vi "Downsample image.vi"(8 "error in (no error)":errorcluster, 10 "Original image":u16[][](array[numeric]), 11 "TomoConversion in":refnum<class "TomoConversion.lvclass">) -> (0 "error out":errorcluster, 2 "Downsampled image":u16[][](array[numeric]), 3 "TomoConversion out":refnum<class "TomoConversion.lvclass">)   [LabVIEW 2012, in "TomoConversion.lvclass"]
uses:
  TomoConversion.lvclass
  TomoConversion.lvclass/TomoConversion.ctl
  <vilib>/Analysis/baseanly.llb/Mean (DBL).vi
  <vilib>/Analysis/NI_AALBase.lvlib
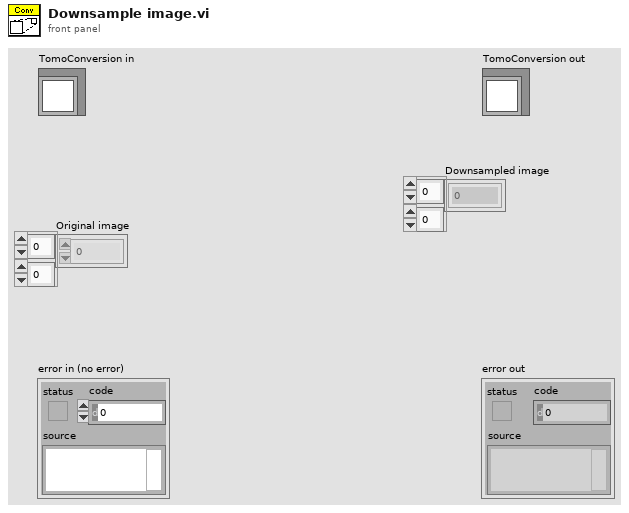
[diagram p1: front panel]
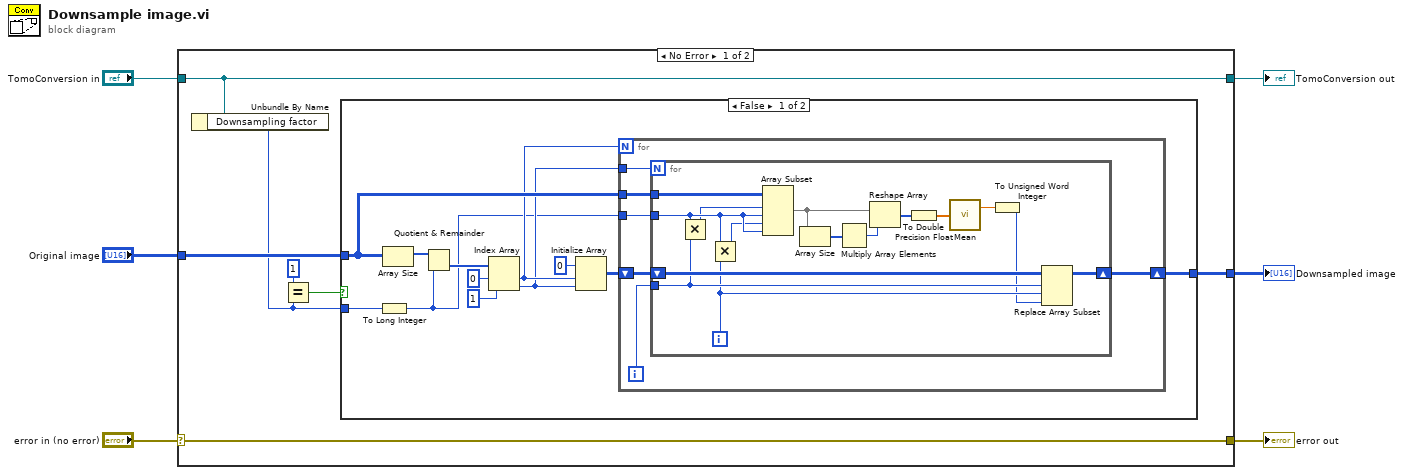
[diagram p0: block diagram]
diagram:
  n1 = case shown="No Error" "error in (no error)" {
    selector: "error in (no error)" -> [w13 w49]
    tunnel: [w13 w49] -> w5
    tunnel: [w8 w48] -> w3
    tunnel: "TomoConversion in" -> [w8 w48]
    tunnel: "Original image" -> [w12 _]
    tunnel: [w11 _] -> w1
    frame No Error {
      n2 = Unbundle By Name(w8) -> ("Downsampling factor"=w7:u32)
      n3 = Equal?(x=u32 1, y=w7) -> (x = y?=w9:bool)
      n4 = case shown="False" w9 {
        tunnel: w7 -> [w24 _]
        tunnel: w12 -> [w18 w47]
        tunnel: [w14 w47] -> w11
        frame False {
          n5 = To Long Integer(number=w24) -> (32bit integer=w15:i32)
          n6 = Array Size(array=w18) -> (size(s)=w25:i32[])
          n7 = Quotient & Remainder(x=w25, y=w15) -> (floor(x/y)=w23:i32[])  [unwired: 1 out]
          n8 = Index Array(array=w23, index #1=0 ("index"), index #2=1 ("index")) -> (element #1=w17:i32, element #2=w16:i32)
          n9 = Initialize Array(u16 0 ("element"), w17, w16) -> (w19:u16[][])
          n10 = for {
            N: w17 -> [_]
            tunnel: w18 -> [w30]
            shift-right: [w26] -> w14
            shift-left: w19 -> [w31]
            tunnel: w16 -> [w28]
            tunnel: w15 -> [w27]
            i -> [w29]
            n11 = for {
              N: w28 -> [_]
              tunnel: w30 -> [w45]
              tunnel: w29 -> [w44]
              shift-right: [w32] -> w26
              shift-left: w31 -> [w46]
              tunnel: w27 -> [w43]
              i -> [w34]
              n12 = Multiply(x=w43, y=w44) -> (x*y=w42:i32)
              n13 = Multiply(x=w43, y=w34) -> (x*y=w41:i32)
              n14 = Array Subset(array=w45, index (row)=w42, length (row)=w43, index (col)=w41, length (col)=w43) -> (w39:u16[][])
              n15 = Array Size(array=w39) -> (size(s)=w40:i32[])
              n16 = Multiply Array Elements(1:w40) -> (0:w38:i32)
              n17 = Reshape Array(w39, w38) -> (w37:u16[])
              n18 = To Double Precision Float(number=w37) -> (double precision float=w36:dbl[])
              n19 = call-poly <vilib>:"Mean.vi"("X"=w36) -> ("mean"=w35:dbl)  [unwired: 1 out]
              n20 = To Unsigned Word Integer(number=w35) -> (unsigned 16bit integer=w33:u16)
              n21 = Replace Array Subset(array=w46, new element=w33, index (row)=w44, index (col)=w34) -> (w32:u16[][])
            }
          }
        }
        frame True {
        }
      }
    }
    frame Error {
    }
  }
  "error out" <- w5
  "TomoConversion out" <- w3
  "Downsampled image" <- w1
